vi "Wiimote Read Data.vi"(7 "Address Space":T1 items=["EEPROM Memory"=0, "Control Register"=4], 8 "error in":errorcluster, 9 "Size":u16, 10 "Offset":u32 format="%06x", 11 "hWiimoteHandle in":u32 format="%08x") -> (0 "error out":errorcluster, 2 "pReportBuffer out":u8[](array[numeric]) format="%02x", 3 "hWiimoteHandle out":u32 format="%08x")   [LabVIEW 2012, in "Wiimote.lvlib"]
uses:
  Wiimote.lvlib
  Wiimote Address Space.ctl
  Wiimote Reporting Mode.ctl
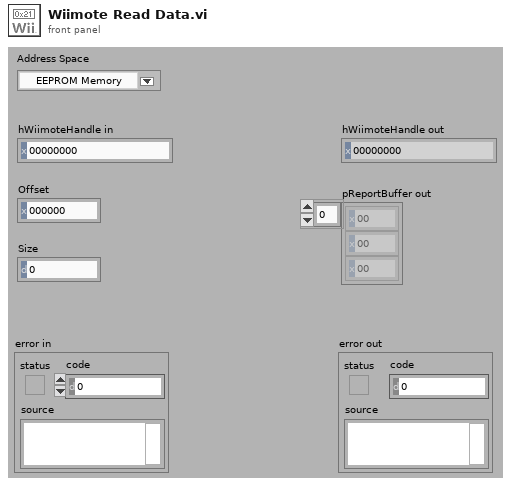
[diagram p1: front panel]
types:
  T1 = typedef "Wiimote.lvlib/Wiimote Address Space.ctl" = u8
  T2 = typedef "Wiimote.lvlib/Wiimote Reporting Mode.ctl" = u8
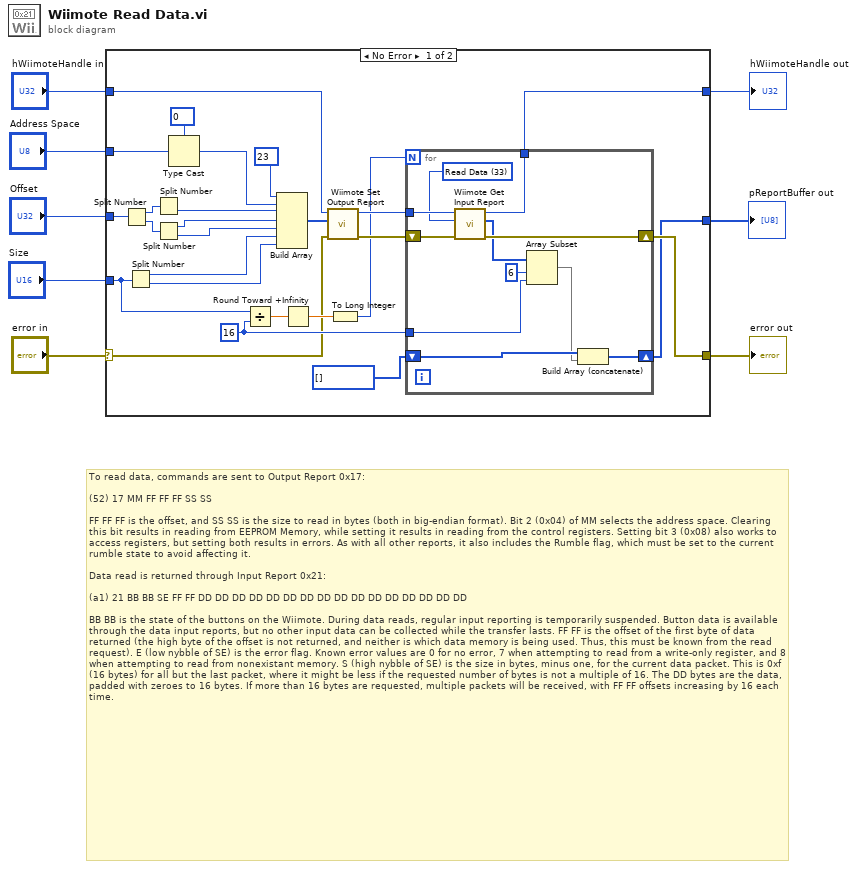
[diagram p0: block diagram]
diagram:
  # "To read data, commands are sent to Output Report 0x17:\n\n(52) 17 MM FF FF FF SS SS\n\nFF FF FF is the offset, and SS SS is the size to read in bytes (both in big-endian format). Bit 2 (0x04) of MM selects the address space. Clearing this bit results in reading from EEPROM Memory, while setting it results in reading from the control registers. Setting bit 3 (0x08) also works to access registers, but setting both results in errors. As with all other reports, it also includes the Rumble flag, which must be set to the current rumble state to avoid affecting it.\n\nData read is returned through Input Report 0x21:\n\n(a1) 21 BB BB SE FF FF DD DD DD DD DD DD DD DD DD DD DD DD DD DD DD DD\n\nBB BB is the state of the buttons on the Wiimote. During data reads, regular input reporting is temporarily suspended. Button data is available through the data input reports, but no other input data can be collected while the transfer lasts. FF FF is the offset of the first byte of data returned (the high byte of the offset is not returned, and neither is which data memory is being used. Thus, this must be known from the read request). E (low nybble of SE) is the error flag. Known error values are 0 for no error, 7 when attempting to read from a write-only register, and 8 when attempting to read from nonexistant memory. S (high nybble of SE) is the size in bytes, minus one, for the current data packet. This is 0xf (16 bytes) for all but the last packet, where it might be less if the requested number of bytes is not a multiple of 16. The DD bytes are the data, padded with zeroes to 16 bytes. If more than 16 bytes are requested, multiple packets will be received, with FF FF offsets increasing by 16 each time."
  n1 = case shown="No Error" "error in" {
    selector: "error in" -> [w9 w46]
    tunnel: [w34 w46] -> w8
    tunnel: "hWiimoteHandle in" -> [w33 w47]
    tunnel: [w32 w47] -> w6
    tunnel: "Offset" -> [w24 _]
    tunnel: "Size" -> [w23 _]
    tunnel: [w22 _] -> w3
    tunnel: "Address Space" -> [w21 _]
    frame No Error {
      w13 = 16 ("y")
      n2 = Split Number(x=w24) -> (hi(x)=w31:u16, lo(x)=w30:u16)
      n3 = Split Number(x=w23) -> (hi(x)=w26:u8, lo(x)=w25:u8)
      n4 = Split Number(x=w31) -> (lo(x)=w28:u8)  [unwired: 1 out]
      n5 = Split Number(x=w30) -> (hi(x)=w27:u8, lo(x)=w29:u8)
      n6 = Type Cast(type=u8 0, x=w21) -> (*(type *) &x=w10:u8)
      n7 = Divide(x=w23, y=w13) -> (x/y=w16:dbl)
      n8 = Build Array(u8 23, w10, w28, w27, w29, w26, w25) -> (w17:u8[])
      n9 = Round Toward +Infinity(x=w16) -> (ceil(x): smallest int >= x=w15:dbl)
      n10 = call "Wiimote Set Output Report.vi"("error in"=w9, "pReportBuffer in"=w17, "hWiimoteHandle in"=w33) -> ("error out"=w19:errorcluster, "hWiimoteHandle out"=w20:u32)  [unwired: 7 in]
      n11 = To Long Integer(number=w15) -> (32bit integer=w14:i32)
      n12 = for {
        N: w14 -> [_]
        tunnel: w20 -> [w45]
        tunnel: [w42] -> w32
        shift-right: [w41] -> w34
        shift-left: w19 -> [w44]
        tunnel: w13 -> [w39]
        shift-right: [w37] -> w22
        shift-left: u8[] [] -> [w38]
        w43 = T2 33 items=["Status Information"=32, "Read Data"=33, "Write Data"=34, "Core Buttons"=48, "Core Buttons and Accelerometer"=49, "Core Buttons with 8 Extension bytes"=50, "Core Buttons and Accelerometer with 12 IR bytes"=51, "Core Buttons with 19 Extension bytes"=52, "Core Buttons and Accelerometer with 16 Extension Bytes"=53, "Core Buttons with 10 IR bytes and 9 Extension Bytes"=54, "Core Buttons and Accelerometer with 10 IR bytes and 6 Extension Bytes"=55] ("bInputReport")
        n13 = call "Wiimote Get Input Report.vi"("error in"=w44, "bInputReport"=w43, "hWiimoteHandle in"=w45) -> ("error out"=w41:errorcluster, "pReportBuffer out"=w35:u8[], "hWiimoteHandle out"=w42:u32)  [unwired: 6 in]
        n14 = Array Subset(array=w35, index=6, length=w39) -> (w36:u8[])
        n15 = Build Array (concatenate)(w38, w36) -> (w37:u8[])
      }
    }
    frame Error {
    }
  }
  "error out" <- w8
  "hWiimoteHandle out" <- w6
  "pReportBuffer out" <- w3
